vi "RT Stream Client.vi"(10 "CamSession":T1="cam0", 11 "Writer url":string="//192.168.11.240/CmdWriter") -> ()   [LabVIEW 2015]
uses:
  Controls/RT Streamer State.ctl
  <vilib>/userdefined/High Color/IMAQdx.ctl
  Controls/RT Streamer Queue element.ctl
  RT Controls/Generic instruction typedef.ctl
  RT Controls/RT Streamer Ack element.ctl
  Controls/Log Thread Name.ctl
  LP Globals.vi
  <vilib>/nisyscfg/Close (System).vi
  <vilib>/nisyscfg/nisyscfg.lvlib
panel:
  out "RT Stream State":T2
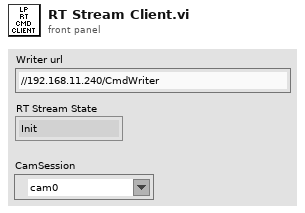
[diagram p1: front panel]
types:
  T1 = typedef "IMAQdx.ctl" = refnum<k21>
  T2 = typedef "RT Streamer State.ctl" = enum16{"Init", "Idle", "Stream", "Listen", "SetRefrashRate", "SendCmdAck", "SendCmdDone", "SendSysState", "StartRecord", "Error"}
  T3 = typedef "RT Streamer Queue element.ctl" = cluster{"CMD":T2, "Data":variant}
  T4 = cluster{"RefreshRate":i32, "ClientRef":refnum<k21>}
  T5 = typedef "Generic instruction typedef.ctl" = cluster{"CMD":string, "Data":variant}
  T6 = typedef "Log Thread Name.ctl" = enum16{"Motor R", "Generic", "Motor P", "Motor Y", "StreamClient", "Stream Server", "Sequencer"}
  T7 = typedef "RT Streamer Ack element.ctl" = cluster{"Data":variant, "CMD":string, "error":errorcluster}
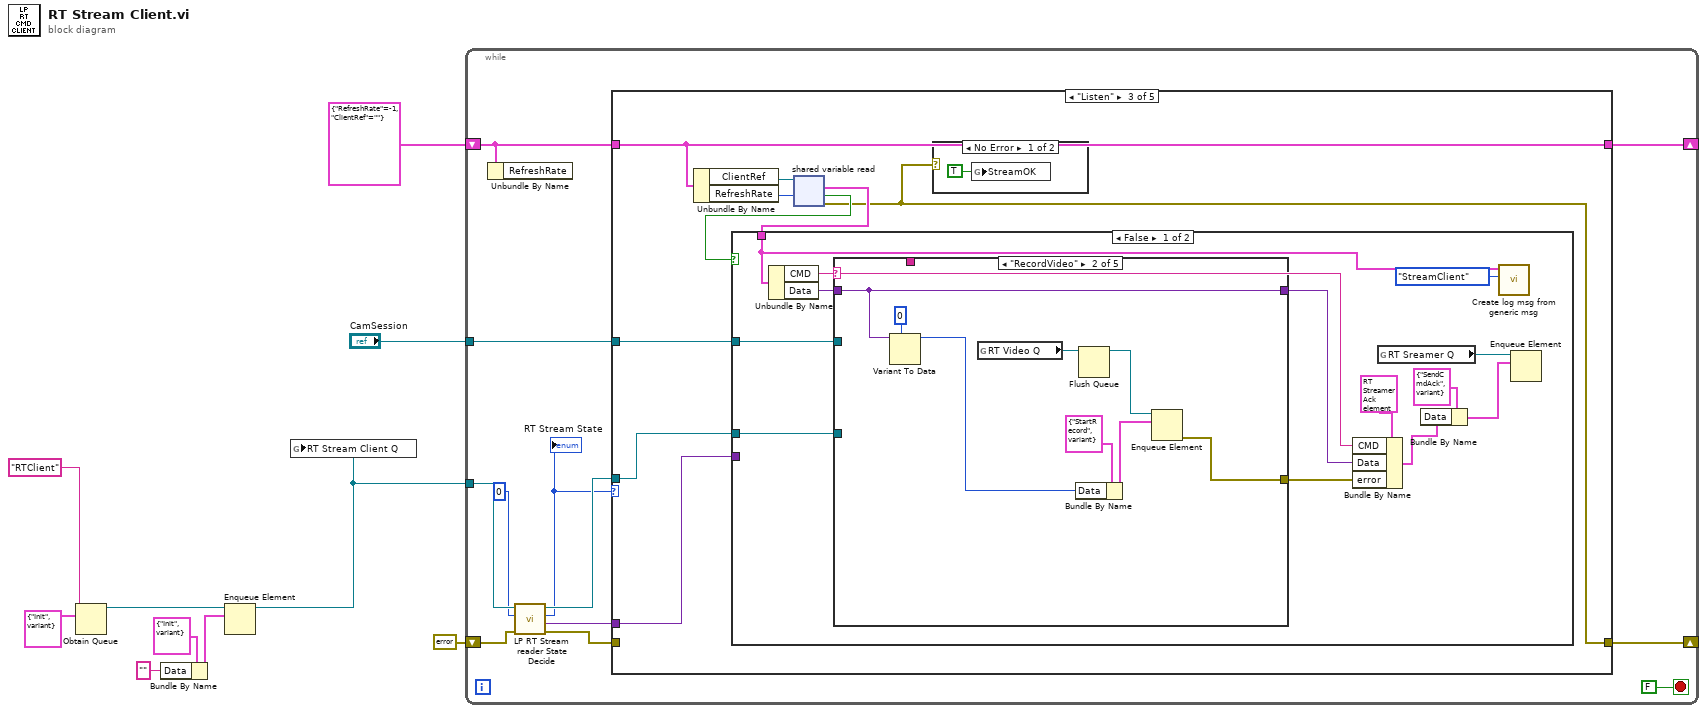
[diagram p0: block diagram]
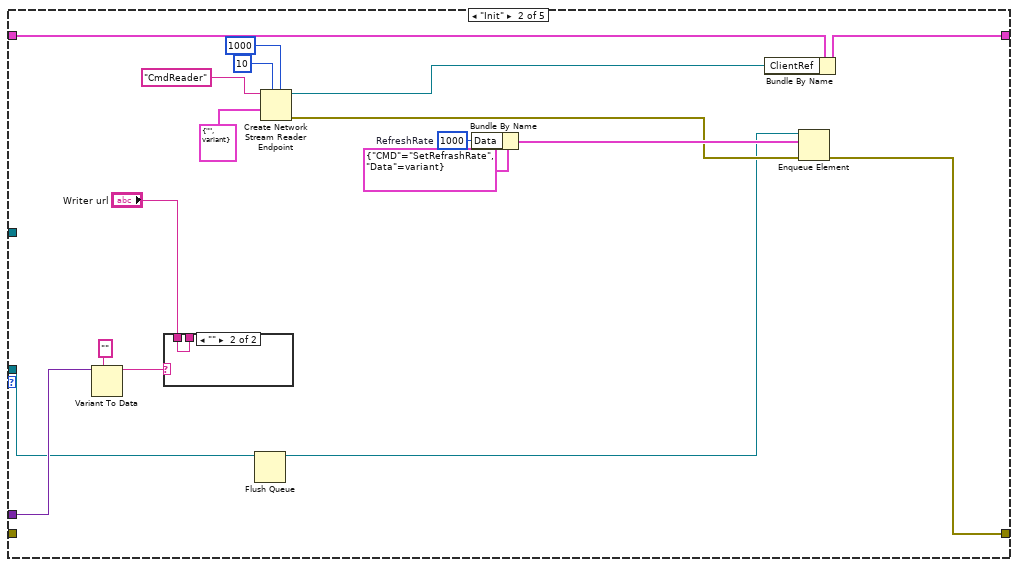
[diagram p3: hidden frame]
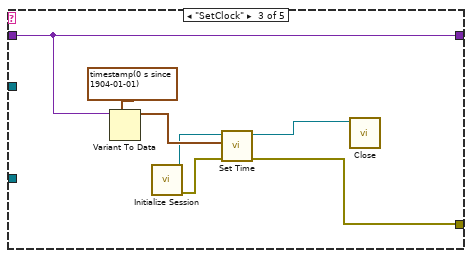
[diagram p7: hidden frame]
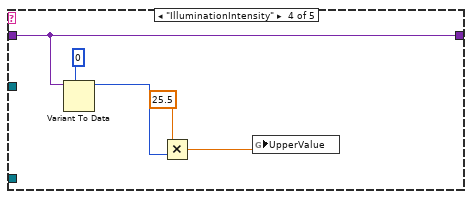
[diagram p8: hidden frame]
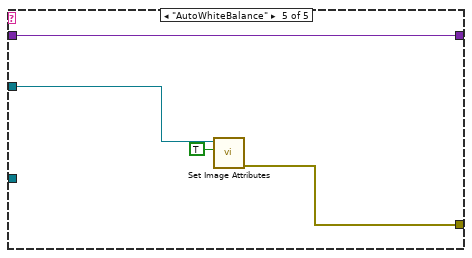
[diagram p9: hidden frame]
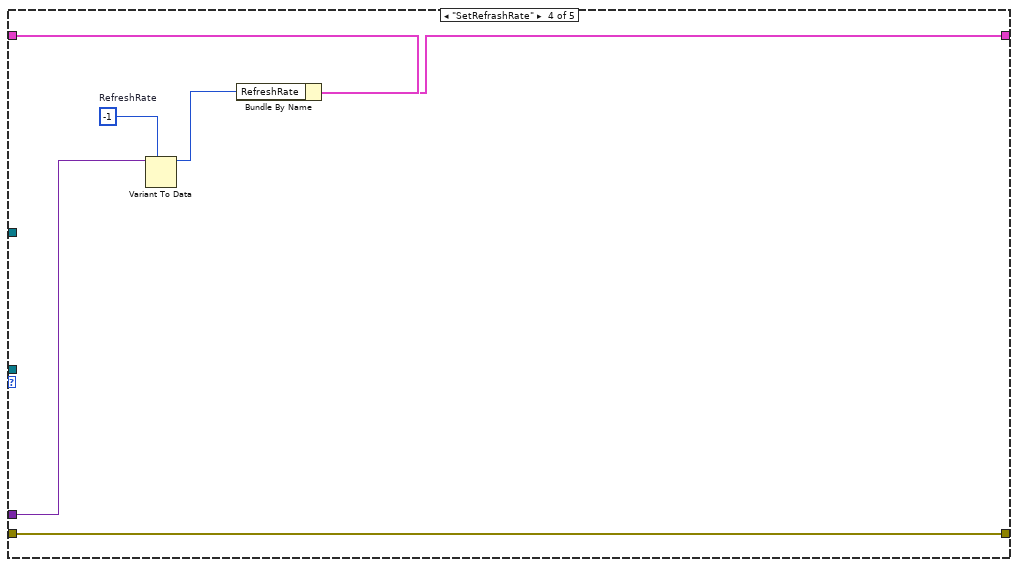
[diagram p11: hidden frame]
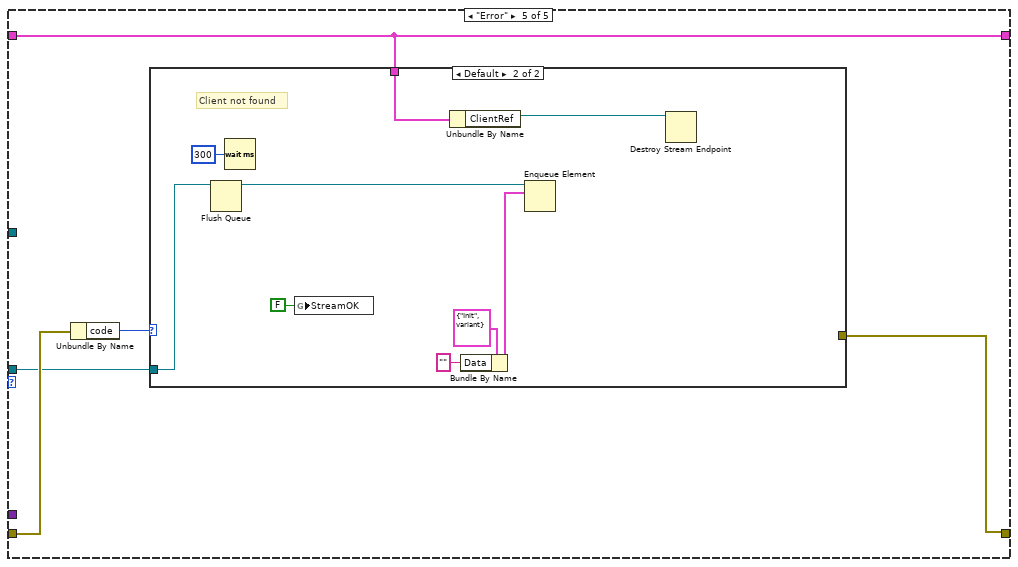
[diagram p12: hidden frame]
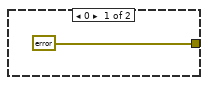
[diagram p13: hidden frame]
diagram:
  n1 = Obtain Queue(name (unnamed)="RTClient", element data type=T3 {"CMD"=enum."Init", "Data"=variant}) -> (queue out=w7:refnum<queue>)  [unwired: 3 in, 2 out]
  n2 = Bundle By Name(cluster=T3 {"CMD"=enum."Init", "Data"=variant} ("element"), "Data"="") -> (w5:T3)
  n3 = Enqueue Element(queue=w7, element=w5) -> (queue out=w2:refnum<queue>)  [unwired: 2 in, 2 out]
  n4 = global write "LP Globals.vi" "RT Stream Client Q"(w2) -> ()
  n5 = while {
    shift-right: [w22] -> _
    shift-left: T4 {"RefreshRate"=-1, "ClientRef"=""} -> [w20]
    shift-right: [w13] -> _
    shift-left: errorcluster {"status"=FALSE, "code"=0, "source"=""} ("error constant") -> [w17]
    tunnel: w2 -> [w19]
    tunnel: "CamSession" -> [w11]
    stop <- FALSE stop-if-true
    n6 = Unbundle By Name(w20) -> ()  [unwired: 1 out]
    n7 = call "LP RT Stream reader State Decide.vi"("error in (no error)"=w17, "RefreshRate"=0, "Queue in"=w19) -> ("error out"=w16:errorcluster, "Data"=w15:variant, "CMD"=w14:T2, "queue out"=w18:refnum<queue>)  [unwired: 5 in]
    "RT Stream State" <- w14
    n8 = case shown="\"Listen\"" w14 {
      tunnel: [w23 w28 w47 w95 w102] -> w13
      tunnel: w20 -> [w24 w41 w53 w97 w100]
      tunnel: [w24 w40 w53 w96 w100] -> w22
      tunnel: w15 -> [_ w39 w48 w99 _]
      tunnel: w16 -> [w23 _ _ w95 w104]
      tunnel: w18 -> [_ w27 w46 _ w101]
      tunnel: w11 -> [_ _ w45 _ _]
      frame "Idle", Default {
      }
      frame "Init" {
        w32 = 1000  # RefreshRate
        n9 = Variant To Data(type="", Variant=w39) -> (data=w37:string)  [unwired: 1 in, 1 out]
        n10 = case shown="\"\"" w37 {
          selector: w37 -> [w43 _]
          tunnel: "Writer url" -> [_ w44]
          tunnel: [w43 w44] -> _
          frame Default {
          }
          frame "" {
          }
        }
        n11 = Flush Queue(queue=w27) -> (queue out=w25:refnum<queue>)  [unwired: 1 in, 2 out]
        n12 = Create Network Stream Reader Endpoint(5:1000 ("timeout in ms (-1)"), 7:10 ("writer buffer size"), 9:T5 {"CMD"="", "Data"=variant}, 11:"CmdReader" ("writer name")) -> (0:w29:errorcluster, 3:w26:refnum<k21>)  [unwired: 3 in]
        n13 = Bundle By Name(cluster=T3 {"CMD"=enum."SetRefrashRate", "Data"=variant} ("element"), "Data"=w32) -> (w31:T3)
        n14 = Bundle By Name(cluster=w41, "ClientRef"=w26) -> (w40:T4)
        n15 = Enqueue Element(queue=w25, element=w31, error in (no error)=w29) -> (error out=w28:errorcluster)  [unwired: 1 in, 2 out]
      }
      frame "Listen" {
        n16 = Unbundle By Name(w53) -> ("ClientRef"=w52:refnum<k21>, "RefreshRate"=w51:i32)
        n17 = shared-variable-read(w52, w51) -> (w47:errorcluster, w50:bool, w49:T5)  [unwired: 1 in, 1 out]
        n18 = case shown="False" w50 {
          tunnel: w49 -> [w59 _]
          tunnel: w48 -> [_ _]
          tunnel: w46 -> [w57 _]
          tunnel: w45 -> [w55 _]
          frame False {
            n19 = Unbundle By Name(w59) -> ("CMD"=w64:string, "Data"=w63:variant)
            n20 = case shown="\"RecordVideo\"" w64 {
              selector: w64 -> [w68 _ _ _ _]
              tunnel: w63 -> [w69 w77 w84 w89 w93]
              tunnel: [w69 w77 w84 w89 w93] -> w60
              tunnel: w57 -> [_ _ _ _ _]
              tunnel: [_ w72 w81 _ w90] -> w56
              tunnel: [w68 _ _ _ _] -> _
              tunnel: w55 -> [_ _ _ _ w92]
              frame Default {
              }
              frame "RecordVideo" {
                n21 = Variant To Data(type=0, Variant=w77) -> (data=w73:i32)  [unwired: 1 in, 1 out]
                n22 = global read "LP Globals.vi" "RT Video Q"() -> (w71:refnum<queue>)
                n23 = Bundle By Name(cluster=T3 {"CMD"=enum."StartRecord", "Data"=variant}, "Data"=w73) -> (w74:T3)
                n24 = Flush Queue(queue=w71) -> (queue out=w70:refnum<queue>)  [unwired: 1 in, 2 out]
                n25 = Enqueue Element(queue=w70, element=w74) -> (error out=w72:errorcluster)  [unwired: 2 in, 2 out]
              }
              frame "SetClock" {
                n26 = Variant To Data(type=timestamp(0 s since 1904-01-01) ("Time"), Variant=w84) -> (data=w82:timestamp)  [unwired: 1 in, 1 out]
                n27 = call <vilib>:"Initialize Session.vi"() -> ("error out"=w78:errorcluster, "Session out"=w80:refnum<k21>)  [unwired: 10 in]
                n28 = call <vilib>:"Set Time.vi"("error in (no error)"=w78, "Time"=w82, "Session in (localhost)"=w80) -> ("error out"=w81:errorcluster, "Session out"=w79:refnum<k21>)  [unwired: 5 in, 2 out]
                n29 = call-poly <vilib>:"Close.vi"("Session in"=w79) -> ()  [unwired: 10 in, 1 out]
              }
              frame "IlluminationIntensity" {
                n30 = Variant To Data(type=0, Variant=w89) -> (data=w86:i32)  [unwired: 1 in, 1 out]
                n31 = Multiply(x=25.5, y=w86) -> (x*y=w85:dbl)
                n32 = global write "LP Globals.vi" "UpperValue"(w85) -> ()
              }
              frame "AutoWhiteBalance" {
                n33 = call "Set Image Attributes.vi"("AutoBalance"=TRUE, "Refnum in"=w92) -> ("error out"=w90:errorcluster)  [unwired: 8 in, 1 out]
              }
            }
            n34 = Bundle By Name(cluster=T7 {"Data"=variant, "CMD"="", "error"={"status"=FALSE, "code"=0, "source"=""}} ("Cluster"), "CMD"=w64, "Data"=w60, "error"=w56) -> (w65:T7)
            n35 = global read "LP Globals.vi" "RT Sreamer Q"() -> (w67:refnum<queue>)
            n36 = Bundle By Name(cluster=T3 {"CMD"=enum."SendCmdAck", "Data"=variant} ("Cluster"), "Data"=w65) -> (w62:T3)
            n37 = call "Create log msg from generic msg.vi"("Thread"=Log_Thread_Name."StreamClient", "variant"=w59) -> ()  [unwired: 10 in]
            n38 = Enqueue Element(queue=w67, element=w62) -> ()  [unwired: 2 in, 3 out]
          }
          frame True {
          }
        }
        n39 = case shown="No Error" w47 {
          frame No Error {
            n40 = global write "LP Globals.vi" "StreamOK"(TRUE ("StreamOK")) -> ()
          }
          frame Error {
          }
        }
      }
      frame "SetRefrashRate" {
        w98 = -1  # RefreshRate
        n41 = Variant To Data(type=w98, Variant=w99) -> (data=w94:i32)  [unwired: 1 in, 1 out]
        n42 = Bundle By Name(cluster=w97, "RefreshRate"=w94) -> (w96:T4)
      }
      frame "Error" {
        n43 = Unbundle By Name(w104) -> ("code"=w103:i32)
        n44 = case shown="Default" w103 {
          tunnel: [errorcluster {"status"=FALSE, "code"=0, "source"=""} ("error constant") _] -> w102
          tunnel: w101 -> [_ w110]
          tunnel: w100 -> [_ w108]
          frame 0 {
          }
          frame Default {
            # "Client not found"
            n45 = Flush Queue(queue=w110) -> (queue out=w109:refnum<queue>)  [unwired: 1 in, 2 out]
            n46 = Wait (ms)(milliseconds to wait=u32 300) -> ()  [unwired: 1 out]
            n47 = global write "LP Globals.vi" "StreamOK"(FALSE ("StreamOK")) -> ()
            n48 = Unbundle By Name(w108) -> ("ClientRef"=w107:refnum<k21>)
            n49 = Bundle By Name(cluster=T3 {"CMD"=enum."Init", "Data"=variant} ("element"), "Data"="") -> (w112:T3)
            n50 = Enqueue Element(queue=w109, element=w112) -> ()  [unwired: 2 in, 3 out]
            n51 = Destroy Stream Endpoint(11:w107) -> ()  [unwired: 1 in, 1 out]
          }
        }
      }
    }
  }
